vi "MU Calibration analyze Raw Data.vi"(7 "numberOfRawDataSamples":u64, 8 "error in (no error)":errorcluster, 9 "noniusTrackRawData":u16[](array[numeric]), 10 "masterTrackRawData":u16[](array[numeric]), 11 "CalibrationHandle":T2) -> (0 "error out (no error)":errorcluster, 3 "CalibrationAnalyzeResultHandle":T1)   [LabVIEW 2017, in "MU_3SL_interface.lvlib"]
uses:
  MU_3SL_interface.lvlib
  handles/CalibrationHandle.ctl
  handles/CalibrationAnalyzeResultHandle.ctl
  lib/MU_3SL_interface.dll
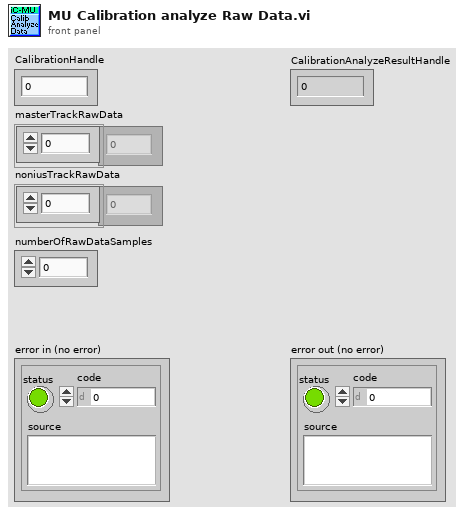
[diagram p1: front panel]
types:
  T1 = typedef "MU_3SL_interface.lvlib/CalibrationAnalyzeResultHandle.ctl" = u64
  T2 = typedef "MU_3SL_interface.lvlib/CalibrationHandle.ctl" = u64
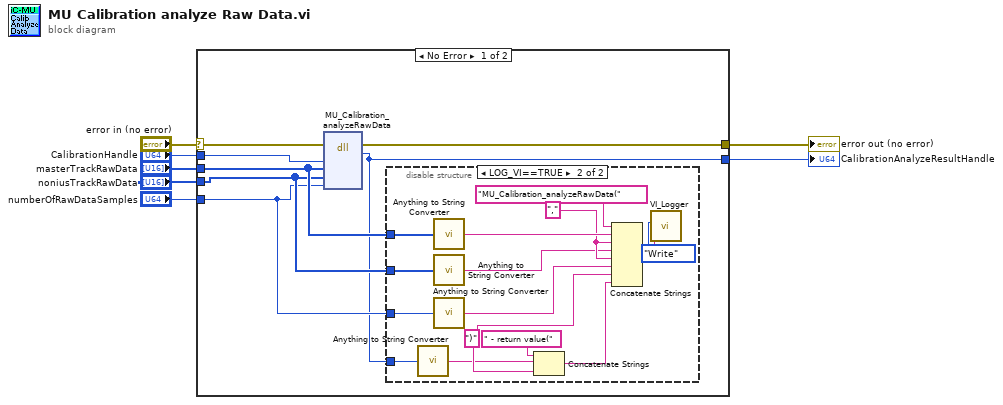
[diagram p0: block diagram]
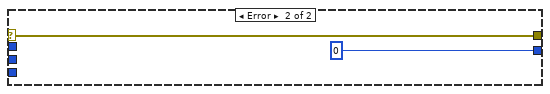
[diagram p3: hidden frame]
diagram:
  n1 = case shown="No Error" "error in (no error)" {
    selector: "error in (no error)" -> [w14 w31]
    tunnel: [w13 w31] -> w7
    tunnel: "CalibrationHandle" -> [w12 _]
    tunnel: [w8 u64 0 ("CalibrationAnalyzeResult")] -> w4
    tunnel: "numberOfRawDataSamples" -> [w9 _]
    tunnel: "masterTrackRawData" -> [w11 _]
    tunnel: "noniusTrackRawData" -> [w10 _]
    frame No Error {
      n2 = dll-call lib="C:/Users/bes/AppData/Roaming/work/mu_9so/icsubmodules/soft_mu_3sl_master/lv_interface/lib/MU_3SL_interface**.*" fn="MU_Calibration_analyzeRawData"(error in=w14, "Calibration"=w12, "masterTrackRawData"=w11, "noniusTrackRawData"=w10, "numberOfRawDataSamples"=w9) -> (error out=w13:errorcluster, "CalibrationAnalyzeResult"=w8:u64)  [unwired: 6 in, 1 out]
      n3 = disable-structure shown="LOG_VI==TRUE" {
        disable-tunnel: w11 -> [_ w25]
        disable-tunnel: w10 -> [_ w22]
        disable-tunnel: w9 -> [_ w20]
        disable-tunnel: w8 -> [_ w15]
        frame condition #0 {
        }
        frame condition #1 (active) {
          w23 = "," ("string")
          w18 = ")" ("string")
          n4 = call "Anything to String Converter.vi"("anything"=w15) -> ("String"=w16:string)
          n5 = call "Anything to String Converter.vi"("anything"=w25) -> ("String"=w24:string)
          n6 = call "Anything to String Converter.vi"("anything"=w22) -> ("String"=w21:string)
          n7 = call "Anything to String Converter.vi"("anything"=w20) -> ("String"=w19:string)
          n8 = Concatenate Strings(" - return value(" ("string"), w16, w18) -> (w17:string)
          n9 = Concatenate Strings("MU_Calibration_analyzeRawData(" ("Info in"), w24, w23, w21, w23, w19, w18, w17) -> (w27:string)
          n10 = call "VI_Logger.vi"("Action (Read)"=enum16{"Write", "Read"}."Write", "Info in"=w27) -> ()  [unwired: 8 in, 2 out]
        }
      }
    }
    frame Error {
    }
  }
  "error out (no error)" <- w7
  "CalibrationAnalyzeResultHandle" <- w4
